vi "write_to_log.vi"(4 "Log":string) -> ()   [LabVIEW 2016]
panel:
  out "error out":errorcluster
  in  "error in":errorcluster
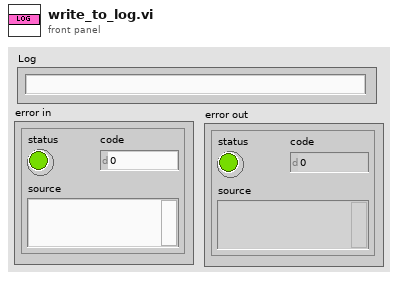
[diagram p1: front panel]
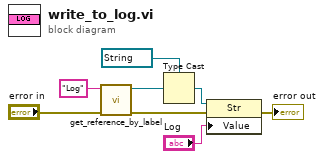
[diagram p0: block diagram]
diagram:
  n1 = call "get_reference_by_label.vi"("error in"="error in", "Label"="Log") -> ("error out"=w3:errorcluster, "Ctl Refnum"=w7:refnum<vi>)  [unwired: 7 in, 1 out]
  n2 = Type Cast(type=refnum<vi> refnum ("Log"), x=w7) -> (*(type *) &x=w5:refnum<vi>)
  n3 = property class="Str"(reference=w5, error in=w3, "Value"="Log") -> (error out=→"error out":errorcluster)  [unwired: 1 out]
